vi "VMI_delays_save_display.vi"(3 "error in":errorcluster, 4 "Save Info":T3={"Collection Information"=[], "ChangeFile"=FALSE, "Image Info"={"X size"=782.0, "Y size"=582.0, "Centroiding"=1.0}, "SAve Paths"=[], "Save"=[], "Current File Date"=""}, 5 "Results":T4, 6 "Delay Number":i32) -> (0 "error out":errorcluster)   [LabVIEW 2019]
uses:
  Type defs/FileAcq_v1_Ctrl.ctl
  Type defs/Image_info.ctl
  Type defs/VMI_peak_out.ctl
panel:
  in  "Remote Save?":bool
  in  "Remote_path":path=path "C:/Users/Parkes/Documents/GitHub/Camera-Acquire_Labview/120416aa"
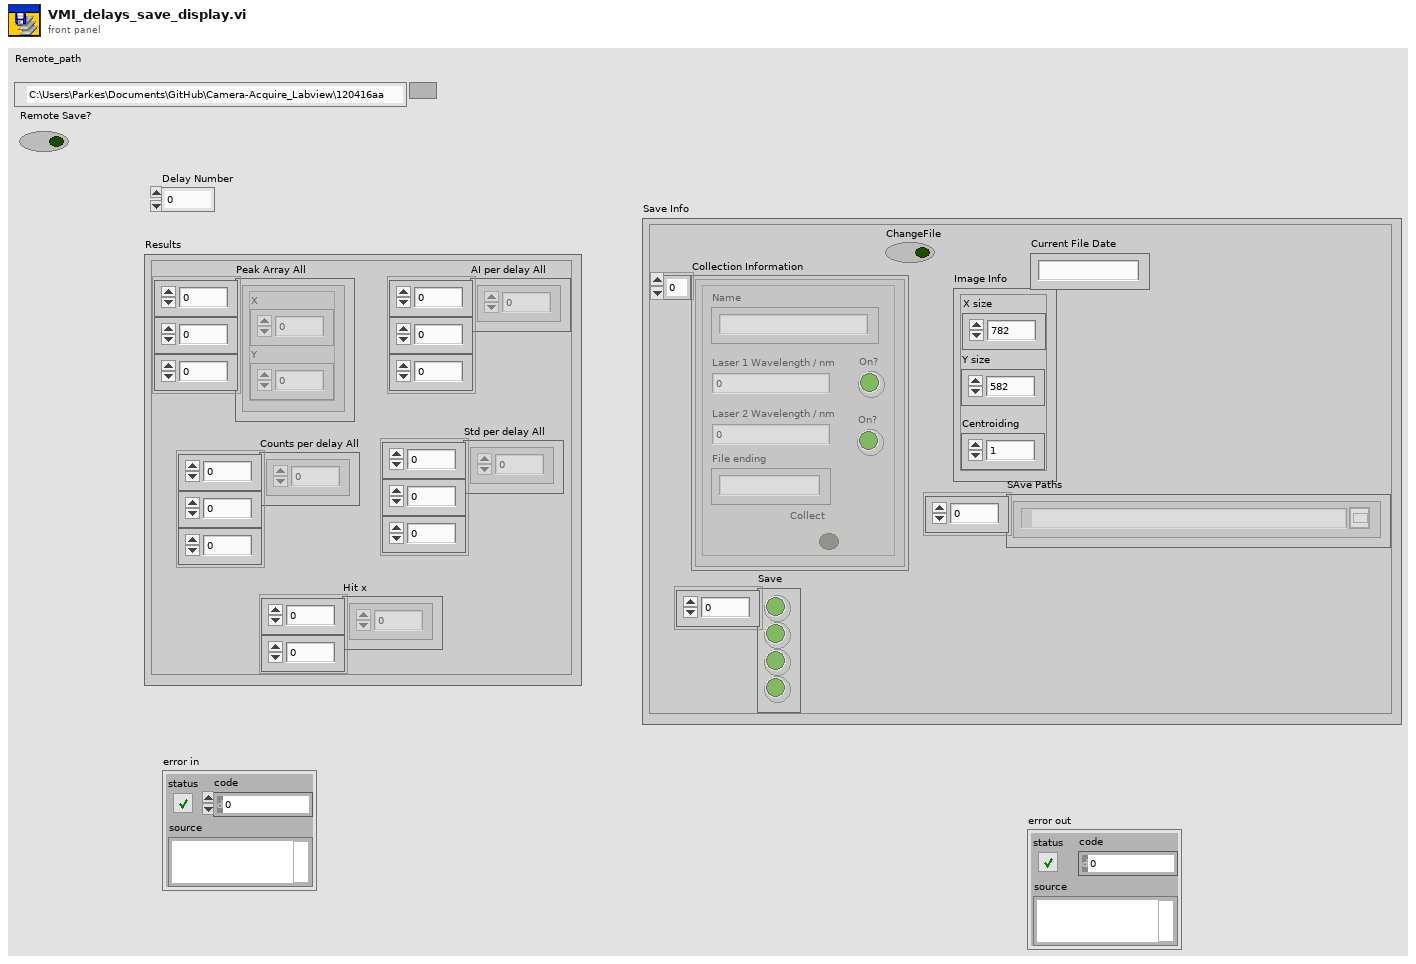
[diagram p1: front panel]
types:
  T1 = typedef "FileAcq_v1_Ctrl.ctl" = cluster{"Type":string, "LaserWave1":dbl, "Shutter1":bool, "LaserWave2":dbl, "Shutter2":bool, "FileEnd":string, "Collect":bool}
  T2 = typedef "Image_info.ctl" = cluster{"X size":dbl, "Y size":dbl, "Centroiding":dbl}
  T3 = cluster{"Collection Information":T1[], "ChangeFile":bool, "Image Info":T2, "SAve Paths":path[], "Save":bool[], "Current File Date":string}
  T4 = cluster{"Peak Array All":cluster{"X":sgl, "Y":sgl}[][][], "AI per delay All":dbl[][][], "Counts per delay All":dbl[][][], "Std per delay All":dbl[][][], "Hit x":dbl[][]}
  T5 = typedef "VMI_peak_out.ctl" = cluster{"Peaks":cluster{"X":sgl, "Y":sgl}[], "size":i32, "Title":string}
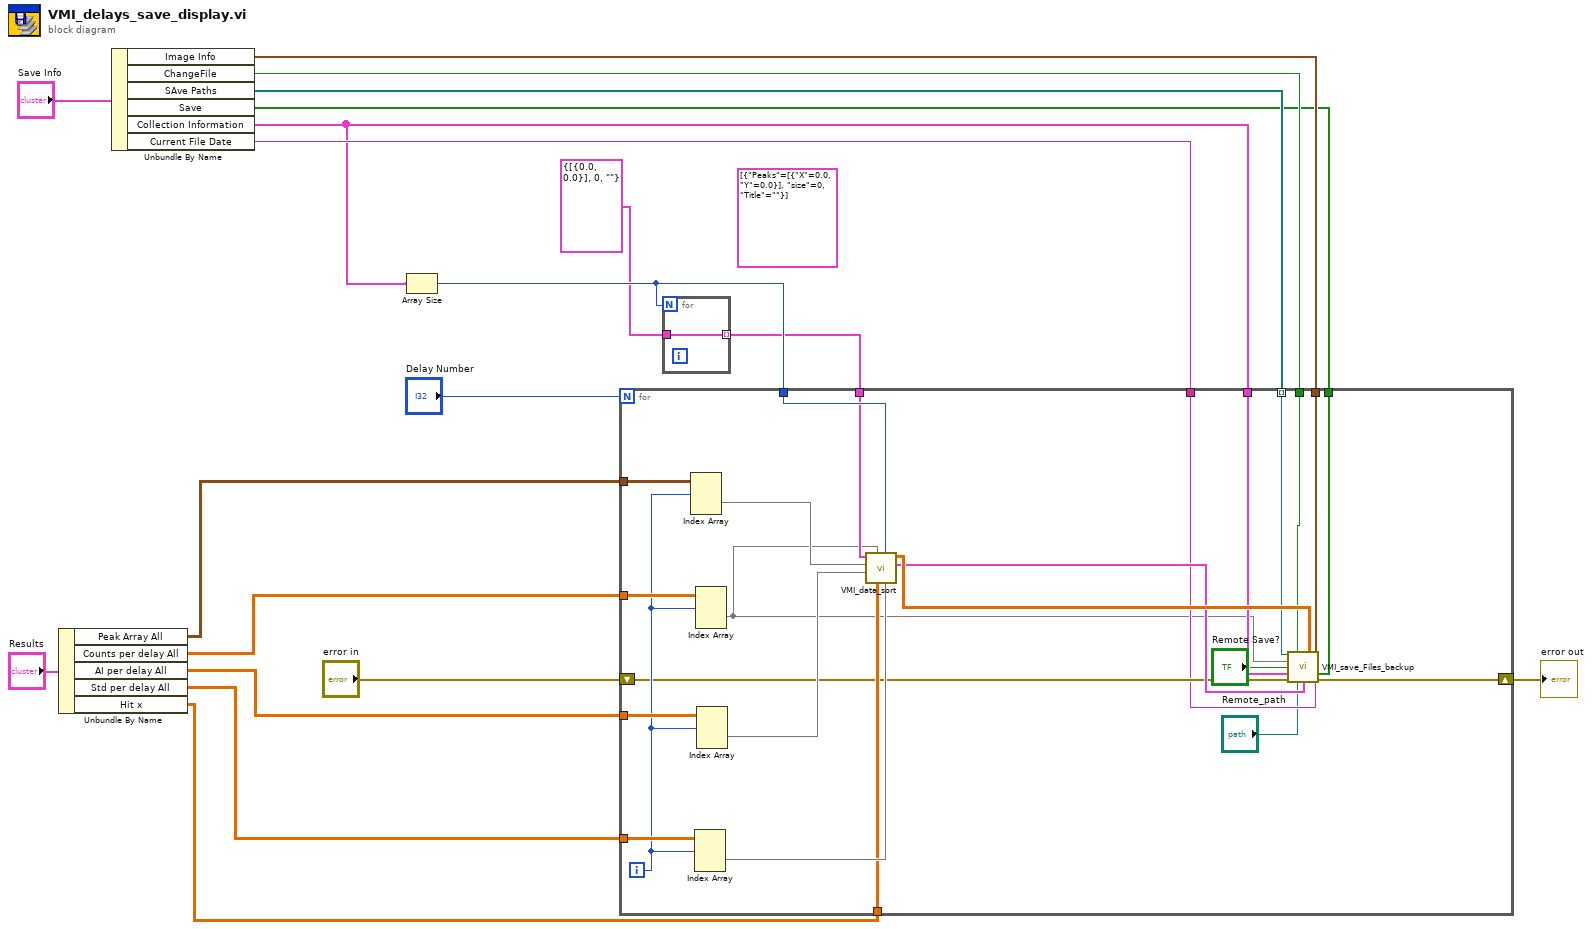
[diagram p0: block diagram]
diagram:
  (unwired) T5[] [{"Peaks"=[{"X"=0.0, "Y"=0.0}], "size"=0, "Title"=""}] ("Data")
  n1 = Unbundle By Name("Results") -> ("Peak Array All"=w15:cluster{"X":sgl, "Y":sgl}[][][], "Counts per delay All"=w14:dbl[][][], "AI per delay All"=w13:dbl[][][], "Std per delay All"=w12:dbl[][][], "Hit x"=w11:dbl[][])
  n2 = Unbundle By Name("Save Info") -> ("Image Info"=w9:T2, "ChangeFile"=w8:bool, "SAve Paths"=w7:path[], "Save"=w6:bool[], "Collection Information"=w4:T1[], "Current File Date"=w5:string)
  n3 = Array Size(array=w4) -> (size(s)=w3:i32)
  n4 = for {
    N: w3 -> [_]
    tunnel: T5 {"Peaks"=[{"X"=0.0, "Y"=0.0}], "size"=0, "Title"=""} ("Peak Controls") -> [w20]
    tunnel: [w20] -> w1 mode=indexing
  }
  n5 = for {
    N: "Delay Number" -> [_]
    tunnel: w15 -> [w44]
    tunnel: w14 -> [w41]
    tunnel: w13 -> [w40]
    tunnel: w12 -> [w38]
    tunnel: w3 -> [w43]
    tunnel: w11 -> [w35]
    tunnel: w1 -> [w34]
    tunnel: w4 -> [w31]
    shift-right: [w30] -> w18
    shift-left: "error in" -> [w29]
    tunnel: w6 -> [w28]
    tunnel: w8 -> [w27]
    tunnel: w9 -> [w26]
    tunnel: w7 -> [w25] mode=indexing
    tunnel: w5 -> [w24]
    i -> [w37]
    n6 = Index Array(array=w44, index (dim 0)=w37) -> (element=w42:cluster{"X":sgl, "Y":sgl}[][])  [unwired: 2 in]
    n7 = Index Array(array=w38, index (dim 0)=w37) -> (element=w36:dbl[][])  [unwired: 2 in]
    n8 = Index Array(array=w41, index (dim 0)=w37) -> (element=w21:dbl[][])  [unwired: 2 in]
    n9 = Index Array(array=w40, index (dim 0)=w37) -> (element=w39:dbl[][])  [unwired: 2 in]
    n10 = call "VMI_data_sort.vi"("Power Err"=w36, "Numeric"=w43, "xaxis"=w35, "Histogram"=w21, "Powers"=w39, "Peak Array"=w42, "Data"=w34) -> ("Data Out"=w32:T5[], "HistArray"=w33:dbl[][][])  [unwired: 3 in]
    n11 = call "VMI_save_Files_backup.vi"("appended path"=w25, "ChangeFile"=w27, "Hist_full"=w33, "Image Info"=w26, "Histogram_array"=w21, "Current File Date"=w24, "Remote Save?"="Remote Save?", "Collection Information"=w31, "Save"=w28, "error in (no error)"=w29, "Remote_path"="Remote_path", "Peaks"=w32) -> ("error out"=w30:errorcluster)  [unwired: 2 in, 1 out]
  }
  "error out" <- w18
